vi "多sheet Excel.vi"() -> ()   [LabVIEW 2014]
uses:
  <vilib>/addons/_office/_exclsub.llb/font.ctl
  <vilib>/Analysis/1siggen.llb/General Periodic Sinc.vi
  <vilib>/addons/_office/excel.llb/Excel Easy Table (num).vi
  <vilib>/Utility/NIReport.llb/NI_report.lvclass
  <vilib>/Utility/NIReport.llb/Excel/NI_Excel.lvclass
  <vilib>/addons/_office/NI_ReportGenerationToolkit.lvlib
  <vilib>/Analysis/NI_AALBase.lvlib
panel:
  out "写入完成":bool
  out "EXCEL路径":path
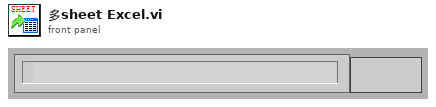
[diagram p1: front panel]
types:
  T1 = enum16{"Standard Report", "HTML", "Word", "Excel"}
  T2 = typedef "NI_ReportGenerationToolkit.lvlib/font.ctl" = cluster{"font name":string, "font size":dbl, "bold":u16, "italic":u16, "underline":u16, "strike through":u16, "font color":u32}
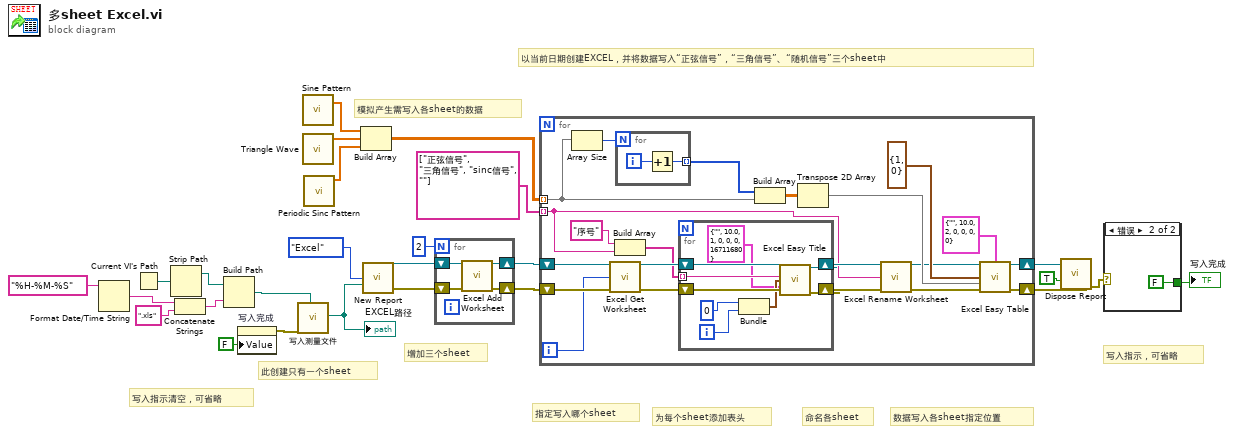
[diagram p0: block diagram]
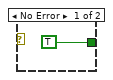
[diagram p2: hidden frame]
diagram:
  # "以当前日期创建EXCEL，并将数据写入“正弦信号”，“三角信号”、“随机信号”三个sheet中"
  # "写入指示，可省略"
  # "写入指示清空，可省略"
  # "命名各sheet"
  # "数据写入各sheet指定位置"
  # "为每个sheet添加表头"
  # "指定写入哪个sheet"
  # "模拟产生需写入各sheet的数据"
  # "增加三个sheet"
  # "此创建只有一个sheet"
  n1 = Format Date/Time String(time format string (%c)="%H-%M-%S" ("时间格式字符串(%c)")) -> (date/time string=w17:string)  [unwired: 2 in]
  n2 = Current VI's Path() -> (path=w15:path)
  n3 = Strip Path(path=w15) -> (stripped path=w14:path)  [unwired: 1 out]
  n4 = Concatenate Strings(w17, ".xls" ("字符串")) -> (w19:string)
  n5 = Build Path(base path=w14, name or relative path=w19) -> (appended path=w11:path)
  n6 = property on="写入完成" class="Bool (严格)"("Value"=FALSE ("写入完成")) -> (error out=w1:errorcluster)  [unwired: 2 in, 1 out]
  n7 = call "写入测量文件"("error in (no error)"=w1, "Filename"=w11) -> ("Filename Out"=w7:path)  [unwired: 15 in, 2 out]
  "EXCEL路径" <- w7
  n8 = call <vilib>:"Sine Pattern.vi"() -> ("Sinusoidal Pattern"=w25:dbl[])  [unwired: 4 in, 1 out]
  n9 = call <vilib>:"Triangle Wave.vi"() -> ("triangle wave"=w24:dbl[])  [unwired: 5 in, 2 out]
  n10 = call <vilib>:"Periodic Sinc Pattern.vi"() -> ("Periodic Sinc Pattern"=w23:dbl[])  [unwired: 10 in, 1 out]
  n11 = Build Array(w25, w24, w23) -> (w9:dbl[][])
  n12 = call <vilib>:"New Report.vi"("report type"=T1."Excel", "template (empty)"=w7) -> ("report out"=w12:refnum<class "NI_report.lvclass">, "error out"=w13:errorcluster)  [unwired: 4 in, 8 out]
  n13 = for {
    N: 2 -> [_]
    shift-right: [w27] -> w2
    shift-left: w13 -> [w30]
    shift-right: [w28] -> w4
    shift-left: w12 -> [w29]
    n14 = call <vilib>:"Excel Add Worksheet.vi"("report in"=w29, "error in (no error)"=w30) -> ("report out"=w28:refnum<class "NI_report.lvclass">, "error out"=w27:errorcluster)  [unwired: 12 in]
  }
  n15 = for {
    tunnel: w9 -> [w36] mode=indexing
    tunnel: string[] ["正弦信号", "三角信号", "sinc信号", ""] -> [w33] mode=indexing
    shift-right: [w46] -> w22
    shift-left: w2 -> [w50]
    shift-right: [w47] -> w21
    shift-left: w4 -> [w51]
    i -> [w38]
    n16 = Array Size(array=w36) -> (size(s)=w37:i32)
    n17 = call <vilib>:"Excel Get Worksheet.vi"("report in"=w51, "worksheet index (0)"=w38, "error in (no error)"=w50) -> ("report out"=w49:refnum<class "NI_report.lvclass">, "error out"=w48:errorcluster)  [unwired: 11 out]
    n18 = Build Array("序号", w33) -> (w32:string[])
    n19 = for {
      N: w37 -> [_]
      tunnel: [w61] -> w35 mode=indexing
      i -> [w62]
      n20 = Increment(x=w62) -> (x+1=w61:i32)
    }
    n21 = for {
      shift-right: [w57] -> w39
      shift-left: w49 -> [w60]
      shift-right: [w58] -> w42
      shift-left: w48 -> [w59]
      tunnel: w32 -> [w56] mode=indexing
      i -> [w54]
      n22 = Bundle(0, w54) -> (w53:cluster{i32, i32})  [unwired: 1 in]
      n23 = call <vilib>:"Excel Easy Title.vi"("report in"=w60, "title"=w56, "start (0, 0)"=w53, "font"=T2 {"font name"="", "font size"=10.0, "bold"=1, "italic"=0, "underline"=0, "strike through"=0, "font color"=16711680}, "error in (no error)"=w59) -> ("report out"=w57:refnum<class "NI_report.lvclass">, "error out"=w58:errorcluster)  [unwired: 1 in, 8 out]
    }
    n24 = Build Array(w35, w36) -> (w43:dbl[][])
    n25 = Transpose 2D Array(2D array=w43) -> (transposed array=w45:dbl[][])
    n26 = call <vilib>:"Excel Rename Worksheet.vi"("report in"=w39, "worksheet name (\"\")"=w33, "error in (no error)"=w42) -> ("report out"=w40:refnum<class "NI_report.lvclass">, "error out"=w41:errorcluster)  [unwired: 11 in]
    n27 = call-poly <vilib>:"Excel Easy Table.vi"("report in"=w40, "font"=T2 {"font name"="", "font size"=10.0, "bold"=2, "italic"=0, "underline"=0, "strike through"=0, "font color"=0}, "start (0, 0)"=cluster{"row":i32, "column":i32} {"row"=1, "column"=0}, "text data"=w45, "error in (no error)"=w41) -> ("report out"=w47:refnum<class "NI_report.lvclass">, "error out"=w46:errorcluster)  [unwired: 4 in, 5 out]
  }
  n28 = call-dynamic "Dispose Report.vi"("report in"=w21, "save changes? (F)"=TRUE, "error in (no error)"=w22) -> ("error out"=w6:errorcluster)  [unwired: 2 in, 10 out]
  n29 = case shown="错误" w6 {
    tunnel: [TRUE FALSE] -> w5
    frame No Error {
    }
    frame Error {
    }
  }
  "写入完成" <- w5
